vi "HFRR ADV v034 new software.vi"() -> ()   [LabVIEW 2025] (continued)
                      }
                      frame #22 {
                        n2405 = Wait (ms)(milliseconds to wait=u32 50) -> ()  [unwired: 1 out]
                      }
                      frame #23 {
                        n2406 = local read "NORMAL LOAD"() -> (w3468:dbl)
                        n2407 = Number To Fractional String(number=w3468, precision (6)=i16 2) -> (F-format string=w3469:string)  [unwired: 2 in]
                        n2408 = Concatenate Strings("Applied Load [grams] :" ("Content"), w3469) -> (w3471:string)
                        n2409 = local read "EVENT LOG"() -> (w3473:string)
                        n2410 = call "Event Log.vi"("Content"=w3471, "EVENT LOG"=w3473) -> ("EVENT LOG"=w3472:string)  [unwired: 8 in, 1 out]
                        n2411 = local write "EVENT LOG"(w3472) -> ()
                      }
                      frame #24 {
                        n2412 = Wait (ms)(milliseconds to wait=u32 50) -> ()  [unwired: 1 out]
                      }
                      frame #25 {
                        n2413 = local read "Set Strk"() -> (w3476:dbl)
                        n2414 = Number To Fractional String(number=w3476, precision (6)=i16 2) -> (F-format string=w3477:string)  [unwired: 2 in]
                        n2415 = Concatenate Strings("Set Stroke [mm] :" ("Content"), w3477) -> (w3479:string)
                        n2416 = local read "EVENT LOG"() -> (w3481:string)
                        n2417 = call "Event Log.vi"("Content"=w3479, "EVENT LOG"=w3481) -> ("EVENT LOG"=w3480:string)  [unwired: 8 in, 1 out]
                        n2418 = local write "EVENT LOG"(w3480) -> ()
                      }
                      frame #26 {
                        n2419 = Wait (ms)(milliseconds to wait=u32 50) -> ()  [unwired: 1 out]
                      }
                      frame #27 {
                        n2420 = local read "Set Temp"() -> (w3484:dbl)
                        n2421 = Number To Fractional String(number=w3484, precision (6)=i16 2) -> (F-format string=w3485:string)  [unwired: 2 in]
                        n2422 = Concatenate Strings("Set Temperature [deg C] :" ("Content"), w3485) -> (w3487:string)
                        n2423 = local read "EVENT LOG"() -> (w3489:string)
                        n2424 = call "Event Log.vi"("Content"=w3487, "EVENT LOG"=w3489) -> ("EVENT LOG"=w3488:string)  [unwired: 8 in, 1 out]
                        n2425 = local write "EVENT LOG"(w3488) -> ()
                      }
                      frame #28 {
                        n2426 = Wait (ms)(milliseconds to wait=u32 50) -> ()  [unwired: 1 out]
                      }
                      frame #29 {
                        n2427 = local read "Set Rh"() -> (w3492:dbl)
                        n2428 = Number To Fractional String(number=w3492, precision (6)=i16 2) -> (F-format string=w3493:string)  [unwired: 2 in]
                        n2429 = Concatenate Strings("Set Humidity [%RH] :" ("Content"), w3493) -> (w3495:string)
                        n2430 = local read "EVENT LOG"() -> (w3497:string)
                        n2431 = call "Event Log.vi"("Content"=w3495, "EVENT LOG"=w3497) -> ("EVENT LOG"=w3496:string)  [unwired: 8 in, 1 out]
                        n2432 = local write "EVENT LOG"(w3496) -> ()
                      }
                      frame #30 {
                        n2433 = Wait (ms)(milliseconds to wait=u32 50) -> ()  [unwired: 1 out]
                      }
                      frame #31 {
                        n2434 = local read "test time"() -> (w3500:dbl)
                        n2435 = Number To Fractional String(number=w3500, precision (6)=i16 1) -> (F-format string=w3501:string)  [unwired: 2 in]
                        n2436 = Concatenate Strings("Test Duration [mins] :" ("Content"), w3501) -> (w3503:string)
                        n2437 = local read "EVENT LOG"() -> (w3505:string)
                        n2438 = call "Event Log.vi"("Content"=w3503, "EVENT LOG"=w3505) -> ("EVENT LOG"=w3504:string)  [unwired: 8 in, 1 out]
                        n2439 = local write "EVENT LOG"(w3504) -> ()
                      }
                      frame #32 {
                        w3506 = dbl[] [] ("History Data")
                        w3507 = cluster{"y":dbl, dbl, "y":dbl}[] [] ("History Data")
                        w3508 = FALSE ("Visible")
                        n2440 = property on="Stroke ( mm )" class="WFChart (strict)"("History Data"=w3507) -> ()  [unwired: 2 in, 2 out]
                        n2441 = property on="Humidity ( %RH )" class="WFChart (strict)"("History Data"=w3506) -> ()  [unwired: 2 in, 2 out]
                        n2442 = property on="Temperature ( Deg C )" class="WFChart (strict)"("History Data"=w3506) -> ()  [unwired: 2 in, 2 out]
                        n2443 = property on="Electrical Contact Resistance ( % )" class="WFChart (strict)"("History Data"=w3506) -> ()  [unwired: 2 in, 2 out]
                        n2444 = property on="Coefficient of Friction" class="WFChart (strict)"("History Data"=w3506) -> ()  [unwired: 2 in, 2 out]
                        n2445 = property on="Frictional Force ( N )" class="WFChart (strict)"("History Data"=w3506) -> ()  [unwired: 2 in, 2 out]
                        n2446 = property on="Coefficient of Friction" class="WFChart (strict)"("History Data"=w3506) -> ()  [unwired: 2 in, 2 out]
                        n2447 = property on="Frictional Force ( N )" class="WFChart (strict)"("History Data"=w3506) -> ()  [unwired: 2 in, 2 out]
                        n2448 = property on="Electrical Contact Resistance ( % )" class="WFChart (strict)"("History Data"=w3506) -> ()  [unwired: 2 in, 2 out]
                        n2449 = property on="Humidity ( %RH )" class="WFChart (strict)"("History Data"=w3506) -> ()  [unwired: 2 in, 2 out]
                        n2450 = property on="Stroke ( mm )" class="WFChart (strict)"("History Data"=w3507) -> ()  [unwired: 2 in, 2 out]
                        n2451 = property on="Temperature ( Deg C )" class="WFChart (strict)"("History Data"=w3506) -> ()  [unwired: 2 in, 2 out]
                        n2452 = property on="Service Password Log" class="Str"("Visible"=w3508) -> ()  [unwired: 2 in, 2 out]
                        n2453 = property on="Password 3" class="Clust (strict)"("Visible"=w3508) -> ()  [unwired: 2 in, 2 out]
                      }
                    }
                    "TEST FILE NAM,E SAVED" <- TRUE ("TEST FILE NAM,E SAVED")
                  }
                }
              }
            }
          }
        }
        n2454 = local write "Test \nStatus"(w2889) -> ()
        n2455 = local write "Save"(w2889) -> ()
        n2456 = local read "Main Tab"() -> (w2883:T2)
        n2457 = case shown="True" w2886 {
          frame False {
            n2458 = local read "Rt 3"() -> (w2958:bool)
            n2459 = case shown="True" w2958 {
              frame False {
              }
              frame True {
                n2460 = local write "Rt 3"(FALSE ("Rt 3")) -> ()
              }
            }
            "Rt" <- TRUE ("Rt")
            "Rt 2" <- FALSE ("Rt")
          }
          frame True {
            n2461 = local read "Rt"() -> (w2964:bool)
            n2462 = local write "Rt 2"(TRUE ("Rt 2")) -> ()
            n2463 = case shown="True" w2964 {
              frame False {
              }
              frame True {
                n2464 = local write "Rt"(FALSE ("Rt")) -> ()
              }
            }
            "Rt 3" <- TRUE ("Rt 3")
          }
        }
        n2465 = case shown="Default" w2883 {
          tunnel: w2885 -> [_ w2993]
          frame Default {
            w2992 = 0.0 ("output")
            n2466 = local write "PID-out"(w2992) -> ()
            n2467 = local write "Frequency ( Hz )"(w2992) -> ()
            n2468 = local write "STROKE Initialize"(TRUE ("STROKE Initialize")) -> ()
          }
          frame "Acquire" {
            n2469 = stacked-sequence {
              frame #0 {
                n2470 = local read "Auto Start Test"() -> (w2995:bool)
                n2471 = case shown="True" w2995 {
                  tunnel: "RUN" -> [w3016 w3019]
                  tunnel: [w3016 w3018] -> w2996
                  frame False {
                  }
                  frame True {
                    n2472 = local read "Auto Start Temp"() -> (w3017:bool)
                    n2473 = Or(x=w3019, y=w3017) -> (x .or. y?=w3018:bool)
                  }
                }
                n2474 = local read "clk"() -> (w3015:dbl)
                n2475 = local read "Save"() -> (w3011:bool)
                n2476 = Equal?(x=w3015, y=0.0) -> (x = y?=w3012:bool)
                n2477 = And(x=w3012, y=w3011) -> (x .and. y?=w3013:bool)
                n2478 = Not(x="Engage") -> (.not. x?=w3002:bool)
                n2479 = case shown="False" w2996 {
                  tunnel: [0.0 w3042] -> w2998
                  frame False {
                    (unwired) TRUE ("Visible")
                    n2480 = local read "Auto Start Test"() -> (w3023:bool)
                    n2481 = local write "Start Time"(TRUE ("Start Time")) -> ()
                    n2482 = property on="Stroke 2" class="DigNum (strict)"("Visible"=FALSE) -> ()  [unwired: 2 in, 2 out]
                    n2483 = case shown="False" w3023 {
                      frame False {
                        n2484 = property on="Heater Button" class="Bool (strict)"("DisabledEnum"=T19."Enabled" ("Disabled")) -> ()  [unwired: 2 in, 2 out]
                        n2485 = property on="Humidity" class="Bool (strict)"("DisabledEnum"=T19."Enabled" ("Disabled")) -> ()  [unwired: 2 in, 2 out]
                      }
                      frame True {
                      }
                    }
                    n2486 = case shown="False" "TestCompFlg" {
                      frame False {
                        n2487 = local read "StartFlg"() -> (w3031:bool)
                        n2488 = case shown="True" w3031 {
                          frame False {
                          }
                          frame True {
                            n2489 = stacked-sequence {
                              frame #0 {
                                n2490 = local read "EVENT LOG"() -> (w3035:string)
                                n2491 = call "Event Log.vi"("Content"="Test was interrupted", "EVENT LOG"=w3035) -> ("EVENT LOG"=w3036:string)  [unwired: 8 in, 1 out]
                                n2492 = local write "EVENT LOG"(w3036) -> ()
                                n2493 = property on="RUN" class="Bool (strict)"("Visible"=TRUE) -> ()  [unwired: 2 in, 2 out]
                                n2494 = property on="Auto Start Test" class="Bool (strict)"("Visible"=TRUE) -> ()  [unwired: 2 in, 2 out]
                              }
                              frame #1 {
                                w3038 = FALSE ("StartFlg")
                                n2495 = property on="Heater Button" class="Bool (strict)"("Val(Sgnl)"=FALSE ("Value (Signaling)")) -> ()  [unwired: 2 in, 2 out]
                                n2496 = local write "Heater Button"(w3038) -> ()
                                n2497 = local write "StartFlg"(w3038) -> ()
                                n2498 = local write "Humidity"(w3038) -> ()
                              }
                              frame #2 {
                                n2499 = local write "Due Write"("VC;0" ("Command")) -> ()
                              }
                              frame #3 {
                                n2500 = Wait (ms)(milliseconds to wait=u32 1500) -> ()  [unwired: 1 out]
                              }
                              frame #4 {
                                n2501 = local write "Due Write"("HE;0" ("Command")) -> ()
                              }
                            }
                          }
                        }
                      }
                      frame True {
                      }
                    }
                    n2502 = local write "String 14"("Test will autostart once parameters reach the set value." ("String 14")) -> ()
                  }
                  frame True {
                    (unwired) FALSE ("Visible")
                    n2503 = property on="Stroke 2" class="DigNum (strict)"("Visible"=TRUE) -> ()  [unwired: 2 in, 2 out]
                    n2504 = property on="STOP 2" class="Bool (strict)"("Disabled"=u8 2) -> ()  [unwired: 2 in, 2 out]
                    n2505 = local write "String 14"(" Running....." ("String 14")) -> ()
                    n2506 = property on="Heater Button" class="Bool (strict)"("DisabledEnum"=T19."Disabled and Grayed Out" ("Disabled")) -> ()  [unwired: 2 in, 2 out]
                    n2507 = property on="Humidity" class="Bool (strict)"("DisabledEnum"=T19."Disabled and Grayed Out" ("Disabled")) -> ()  [unwired: 2 in, 2 out]
                    n2508 = case shown="True" "Start Time" {
                      selector: "Start Time" -> [_ w3061]
                      frame False {
                      }
                      frame True {
                        n2509 = Not(x=w3061) -> (.not. x?=w3060:bool)
                        n2510 = local write "Start Time"(w3060) -> ()
                        n2511 = local read "EVENT LOG"() -> (w3062:string)
                        n2512 = call "Event Log.vi"("Content"="Test in progress", "EVENT LOG"=w3062) -> ("EVENT LOG"=w3064:string)  [unwired: 8 in, 1 out]
                        n2513 = local write "EVENT LOG"(w3064) -> ()
                      }
                    }
                    n2514 = disable-structure shown="Enabled" {
                      disable-tunnel: [w3053 w3059] -> w3042
                      frame Disabled {
                        n2515 = local read "Set Hz"() -> (w3056:dbl)
                        n2516 = call <vilib>:"Uniform White Noise Waveform.vi"() -> ("signal out"=w3055:waveform(dbl))  [unwired: 10 in, 1 out]
                        n2517 = Random Number (0-1)() -> (number: 0 to 1=w3052:dbl)
                        n2518 = Add(x=w3056, y=w3055) -> (x+y=w3054:waveform(dbl))
                        n2519 = Multiply(x=ext 0.01 ("y"), y=w3052) -> (x*y=w3050:ext)
                        n2520 = Multiply(x=w3054, y=w3050) -> (x*y=w3053:waveform(ext))
                      }
                      frame Enabled {
                        n2521 = call-poly <vilib>:"Random Number (Range).vi"("lower bound (0)"=49.89, "upper bound (100)"=50.8) -> ("number"=w3059:dbl)  [unwired: 9 in]
                      }
                    }
                    "StartFlg" <- TRUE ("StartFlg")
                  }
                }
                n2522 = case shown="True" w3013 {
                  frame False {
                  }
                  frame True {
                    n2523 = local write "clk"(10.0 ("clk")) -> ()
                    n2524 = Get Date/Time In Seconds() -> (seconds since 1Jan1904=w3067:timestamp)
                    n2525 = To Double Precision Float(number=w3067) -> (double precision float=w3065:dbl)
                    n2526 = local write "acq timer"(w3065) -> ()
                    n2527 = local write "act save time"(w3065) -> ()
                  }
                }
                n2528 = call "Elapsed Time"("Time Target (s)"="Countdown", "Reset"=w3002) -> ("Elapsed Time (s)"=w3007:dbl, "Time has Elapsed"=w3005:bool)  [unwired: 10 in, 6 out]
                "Countdown 2" <- w3007
                n2529 = Subtract(x=w3007, y=2.0) -> (x-y=w3010:dbl)
                n2530 = Less?(x=w3010, y="Countdown") -> (x < y?=w3008:bool)
                n2531 = And(x=w3008, y=w3005) -> (x .and. y?=w3004:bool)
                n2532 = case shown="True" w3004 {
                  frame False {
                  }
                  frame True {
                    (unwired) dbl[] [] ("History Data")
                    n2533 = local write "Engage"(FALSE ("Engage")) -> ()
                    n2534 = local write "RUN"(TRUE ("RUN")) -> ()
                    n2535 = local read "Humidity ( %RH )"() -> (→"Rh Before":dbl)
                  }
                }
                n2536 = local read "Test \nStatus"() -> (w3000:bool)
                n2537 = Select(t=w2998, s=w3000, f=0.0) -> (s? t:f=w2999:dbl)
                n2538 = local write "Frequency ( Hz )"(w2999) -> ()
              }
              frame #1 {
                w3090 = 1000000.0 ("x")
                # "HC;1/0\nST;VALUE"
                # "Elapsed time\ncof\nstroke\nAir temp\nTemp\nHumidity"
                # "acq timer\n\nact save time"
                # "convert to microseconds"
                n2539 = local read "COUNT"() -> (w3073:i32)
                n2540 = local read "Rate"() -> (w3086:dbl)
                n2541 = Divide(x=w3090, y=w3086) -> (x/y=w3091:dbl)
                n2542 = Greater Or Equal?(x=w3073, y=250) -> (x >= y?=w3072:bool)
                n2543 = Get Date/Time In Seconds() -> (seconds since 1Jan1904=w3093:timestamp)
                n2544 = case shown="True" w3072 {
                  frame False {
                    n2545 = local read "COUNT"() -> (w3094:i32)
                    n2546 = Increment(x=w3094) -> (x+1=w3095:i32)
                    n2547 = local write "COUNT"(w3095) -> ()
                  }
                  frame True {
                    n2548 = local write "COUNT"(0 ("COUNT")) -> ()
                  }
                }
                n2549 = local read "Samplingtime 2"() -> (w3071:dbl)
                n2550 = local read "act save time"() -> (w3088:dbl)
                n2551 = Divide(x=w3091, y=w3090) -> (x/y=w3089:dbl)
                n2552 = To Double Precision Float(number=w3093) -> (double precision float=w3082:dbl)
                n2553 = Add(x=w3088, y=w3071) -> (x+y=w3087:dbl)
                n2554 = local read "acq timer"() -> (w3092:dbl)
                n2555 = local read "COUNT"() -> (w3075:i32)
                n2556 = Greater Or Equal?(x=w3082, y=w3087) -> (x >= y?=w3070:bool)
                n2557 = Multiply(x=w3089, y=w3075) -> (x*y=w3081:dbl)
                n2558 = Subtract(x=w3082, y=w3092) -> (x-y=w3084:dbl)
                n2559 = local read "Save"() -> (w3085:bool)
                n2560 = Add(x=w3084, y=w3081) -> (x+y=w3068:dbl)
                "Elapsed time 3" <- w3068
                n2561 = And(x=w3070, y=w3085) -> (x .and. y?=w3083:bool)
                n2562 = Divide(x=w3068, y=60.0) -> (x/y=w3079:dbl)
                n2563 = local read "Test \nStatus"() -> (w3069:bool)
                n2564 = local read "clk"() -> (w3076:dbl)
                n2565 = Equal?(x=w3076, y=10.0) -> (x = y?=w3078:bool)
                n2566 = case shown="True" w3083 {
                  tunnel: w3082 -> [_ w3208]
                  tunnel: [FALSE ("Boolean 2") TRUE ("Boolean 2")] -> _
                  frame False {
                  }
                  frame True {
                    w3162 = ";" ("Substring")
                    # "Pid out/\nFreq response value"
                    n2567 = local write "act save time"(w3208) -> ()
                    n2568 = local read "FILE"() -> (w3156:string)
                    n2569 = call "file check.vi"("file name in"=w3156) -> ("error out"=w3159:errorcluster, "file name out"=w3154:string)  [unwired: 9 in]
                    n2570 = local read "LVDT STROKE"() -> (w3151:dbl)
                    n2571 = local read "Add up Stroke"() -> (w3149:dbl)
                    n2572 = call "FILE PATH CREATION.vi"("error in"=w3159, "FILE NAME :"=w3154) -> ("FILE OUT"=w3157:path)  [unwired: 8 in, 1 out]
                    n2573 = local read "STROKE Initialize"() -> (w3144:bool)
                    n2574 = Concatenate Strings(w3154, ".dgf" ("Substring")) -> (w3158:string)
                    n2575 = Subtract(x=w3151, y=w3149) -> (x-y=w3150:dbl)
                    n2576 = Absolute Value(x=w3150) -> (abs(x)=w3147:dbl)
                    n2577 = local read "FF 2"() -> (→"Frictional Force ( N )" →"Frictional Force ( N )":dbl)
                    n2578 = Build Path(base path=w3157, name or relative path=w3158) -> (appended path=w3153:path)
                    n2579 = flat-sequence {
                      tunnel: w3147 -> [w3213]
                      tunnel: [w3212] -> w3145
                      tunnel: w3144 -> [w3210]
                      tunnel: [w3215] -> w3146
                      tunnel: w3145 -> [w3215]
                      frame #0 {
                        n2580 = call <vilib>:"Mean PtByPt.vi"("x"=w3213, "sample length"="STROKE FILTER", "initialize"=w3210) -> ("mean"=w3212:dbl)  [unwired: 1 in, 1 out]
                      }
                      frame #1 {
                        "STROKE Initialize" <- FALSE ("STROKE Initialize")
                      }
                    }
                    n2581 = local read "COF 2"() -> (w3167:dbl)
                    "Coefficient of Friction" <- w3167
                    "COF 4" <- w3167
                    "Coefficient of Friction" <- w3167
                    n2582 = local read "TEMP"() -> (w3170:dbl)
                    "Temperature ( Deg C )" <- w3170
                    n2583 = local read "Humidity ( %RH )"() -> (w3169:dbl)
                    "Humidity ( %RH )" <- w3169
                    "Humidity ( %RH )" <- w3169
                    n2584 = local read "Frequency ( Hz )"() -> (w3176:dbl)
                    n2585 = local read "LVDT STROKE DISPLAY"() -> (w3148:dbl)
                    n2586 = local read "Elapsed time"() -> (w3201:dbl)
                    n2587 = local read "AIR TEMP"() -> (w3174:dbl)
                    n2588 = local read "PID-out"() -> (w3179:dbl)
                    n2589 = local write "Temperature ( Deg C )"(w3170) -> ()
                    n2590 = Number To Fractional String(number=w3148, width (-)=i16 9 ("precision (6)"), precision (6)=i16 6) -> (F-format string=w3194:string)  [unwired: 1 in]
                    n2591 = Number To Fractional String(number=w3174, width (-)=i16 9 ("precision (6)"), precision (6)=i16 3) -> (F-format string=w3193:string)  [unwired: 1 in]
                    n2592 = Number To Fractional String(number=w3170, width (-)=i16 9 ("precision (6)"), precision (6)=i16 3) -> (F-format string=w3190:string)  [unwired: 1 in]
                    n2593 = Number To Fractional String(number=w3169, width (-)=i16 9 ("precision (6)"), precision (6)=i16 3) -> (F-format string=w3187:string)  [unwired: 1 in]
                    n2594 = Number To Fractional String(number=0.0, width (-)=i16 9 ("precision (6)"), precision (6)=i16 3) -> (F-format string=w3184:string)  [unwired: 1 in]
                    n2595 = Number To Fractional String(number=w3179, width (-)=i16 9 ("precision (6)"), precision (6)=i16 3) -> (F-format string=w3180:string)  [unwired: 1 in]
                    n2596 = Number To Fractional String(number=w3176, width (-)=i16 9 ("precision (6)"), precision (6)=i16 3) -> (F-format string=w3175:string)  [unwired: 1 in]
                    n2597 = Number To Fractional String(number=w3167, width (-)=i16 9 ("precision (6)"), precision (6)=i16 6) -> (F-format string=w3202:string)  [unwired: 1 in]
                    n2598 = Number To Fractional String(number=w3201, width (-)=i16 14 ("precision (6)"), precision (6)=i16 3) -> (F-format string=w3203:string)  [unwired: 1 in]
                    n2599 = Bundle("y"=1.02, "LVDT STROKE DISPLAY"=w3148, "y"=0.98) -> (w3168:T30)  [unwired: 1 in]
                    n2600 = Number To Fractional String(number="Ambient Humidity :", width (-)=i16 9 ("precision (6)"), precision (6)=i16 6) -> (F-format string=w3160:string)  [unwired: 1 in]
                    n2601 = local read "RUN"() -> (w3166:bool)
                    n2602 = case shown="True" w3166 {
                      tunnel: w3168 -> [_ w3219]
                      tunnel: w3148 -> [_ w3218]
                      tunnel: w3148 -> [_ w3216]
                      tunnel: w3148 -> [_ w3217]
                      frame False {
                      }
                      frame True {
                        "Stroke ( mm )" <- w3219
                        "Stroke ( mm )" <- w3219
                        "Stroke 4" <- w3218
                        "Stroke 3" <- w3216
                        "Stroke 2" <- w3217
                        "measured_stroke" <- w3216
                      }
                    }
                    n2603 = Concatenate Strings(w3203, w3162, w3202, w3162, w3194, w3162, w3193, w3162, w3190, w3162, w3187, w3162, w3184, w3162, w3180, w3162, w3175, w3162, w3160, "\r") -> (w3200:string)
                    n2604 = call <vilib>:"Write Characters To File.vi"("append to file? (new file:F)"=TRUE, "character string"=w3200, "file path (dialog if empty)"=w3153) -> ()  [unwired: 2 in, 1 out]
                    "refresh flag" <- TRUE ("refresh flag")
                    "LVDT STROKE Actual" <- w3146
                  }
                }
                n2605 = case shown="True" w3069 {
                  tunnel: w3079 -> [_ w3105]
                  tunnel: w3084 -> [_ w3115]
                  tunnel: [0.0 w3111] -> _
                  tunnel: w3078 -> [_ w3110]
                  tunnel: [0.0 w3109] -> _
                  tunnel: w3068 -> [_ w3109]
                  tunnel: w3082 -> [w3098 _]
                  frame False {
                    n2606 = local write "acq timer"(w3098) -> ()
                    n2607 = local write "Test Duration Status"(0.0 ("Test Duration Status")) -> ()
                  }
                  frame True {
                    n2608 = local read "Set Hz"() -> (w3112:dbl)
                    n2609 = local write "Elapsed time"(w3105) -> ()
                    n2610 = local read "test time"() -> (w3104:dbl)
                    n2611 = Multiply(x=w3115, y=w3112) -> (x*y=w3114:dbl)
                    n2612 = case shown="False" w3110 {
                      tunnel: w3114 -> [w3116 _]
                      tunnel: [w3116 1.0] -> w3111
                      frame False {
                        n2613 = local write "Cycles elapsed"(w3116) -> ()
                      }
                      frame True {
                      }
                    }
                    n2614 = Greater?(x=w3105, y=w3104) -> (0:w3113:bool)
                    n2615 = Subtract(x=w3104, y=w3105) -> (x-y=w3103:dbl)
                    n2616 = Multiply(x=w3103, y=60.0) -> (x*y=w3102:dbl)
                    n2617 = local write "Time Remaining"(w3102) -> ()
                    n2618 = local write "Remaining Time"(w3102) -> ()
                    n2619 = case shown="True" w3113 {
                      frame False {
                      }
                      frame True {
                        n2620 = stacked-sequence {
                          frame #0 {
                            w3121 = T19."Enabled" ("Disabled")
                            w3120 = FALSE ("TEST FILE NAM,E SAVED")
                            w3122 = "" ("FILE")
                            w3123 = TRUE ("Visible")
                            n2621 = local write "Humidity"(FALSE ("Humidity")) -> ()
                            n2622 = local write "RUN"(FALSE ("OK Button 2")) -> ()
                            n2623 = local write "Heater Button"(FALSE ("Heater Button")) -> ()
                            n2624 = local write "Auto Start Test"(FALSE ("Auto Start Test")) -> ()
                            n2625 = local write "TestCompFlg"(TRUE ("StpFlg")) -> ()
                            n2626 = local read "Humidity ( %RH )"() -> (→"Rh After":dbl)
                            n2627 = property on="STOP 2" class="Bool (strict)"("Disabled"=u8 0) -> ()  [unwired: 2 in, 2 out]
                            n2628 = local read "EVENT LOG"() -> (w3128:string)
                            n2629 = call "Event Log.vi"("Content"="Test Completed", "EVENT LOG"=w3128) -> ("EVENT LOG"=w3127:string)  [unwired: 8 in, 1 out]
                            n2630 = property on="RUN" class="Bool (strict)"("Visible"=w3123) -> ()  [unwired: 2 in, 2 out]
                            n2631 = property on="Auto Start Test" class="Bool (strict)"("Visible"=w3123) -> ()  [unwired: 2 in, 2 out]
                            n2632 = local write "Batch Ref Num :"(w3122) -> ()
                            n2633 = local write "FILE"(w3122) -> ()
                            n2634 = local write "EVENT LOG"(w3127) -> ()
                            n2635 = local write "TEST FILE NAM,E SAVED"(w3120) -> ()
                            n2636 = local write "Fuel Discription :"(w3122) -> ()
                            n2637 = local write "START TEMP"(w3120) -> ()
                            n2638 = local write "Remarks :"(w3122) -> ()
                            n2639 = local write "Main Dashboard Buttons"(T1."Imaging" ("Main Dashboard Buttons")) -> ()
                            n2640 = local write "Main Tab"(T2."Adv Scar" ("Main Tab")) -> ()
                            n2641 = property on="FRICVALZ 2" class="Bool (strict)"("DisabledEnum"=w3121) -> ()  [unwired: 2 in, 2 out]
                            n2642 = property on="FRICVALZ 3" class="Bool (strict)"("DisabledEnum"=w3121) -> ()  [unwired: 2 in, 2 out]
                            n2643 = property on="FRICVALZ 4" class="Bool (strict)"("DisabledEnum"=w3121) -> ()  [unwired: 2 in, 2 out]
                          }
                          frame #1 {
                            n2644 = Wait (ms)(milliseconds to wait=u32 1500) -> ()  [unwired: 1 out]
                          }
                          frame #2 {
                            n2645 = local write "Due Write"("VC;0") -> ()
                          }
                          frame #3 {
                            n2646 = Wait (ms)(milliseconds to wait=u32 1500) -> ()  [unwired: 1 out]
                          }
                          frame #4 {
                            n2647 = local write "Due Write"("VC;0") -> ()
                          }
                          frame #5 {
                            n2648 = Wait (ms)(milliseconds to wait=u32 1500) -> ()  [unwired: 1 out]
                          }
                          frame #6 {
                            n2649 = local write "Due Write"("ST;0") -> ()
                          }
                          frame #7 {
                            n2650 = local write "measured_stroke"(0.0 ("measured_stroke")) -> ()
                            n2651 = Wait (ms)(milliseconds to wait=u32 1500) -> ()  [unwired: 1 out]
                          }
                          frame #8 {
                            n2652 = local write "Due Write"("HE;0") -> ()
                          }
                        }
                      }
                    }
                    n2653 = Divide(x=w3105, y=w3104) -> (x/y=w3108:dbl)
                    n2654 = Multiply(x=w3108, y=100.0) -> (x*y=w3106:dbl)
                    n2655 = local write "Test Duration Status"(w3106) -> ()
                  }
                }
              }
              frame #2 {
                n2656 = case shown="True" "Heater Button" {
                  tunnel: [0.0 ("output") w3242] -> w3220
                  frame False {
                    w3223 = TRUE ("tmpchk")
                    n2657 = local read "TEMP"() -> (w3224:dbl)
                    n2658 = local write "Temp ini"(w3224) -> ()
                    n2659 = local write "Reset 4"(w3223) -> ()
                    n2660 = local write "tmpchk"(w3223) -> ()
                    n2661 = local write "reinit"(TRUE ("reinit")) -> ()
                    n2662 = local write "manual temp log"(TRUE ("manual temp log")) -> ()
                  }
                  frame True {
                    # "Logic to turn off\nthe heater when \ntemp is not rising.\nTime - 60 sec\nDelta t- 5°c"
                    n2663 = local read "Temp ini"() -> (w3231:dbl)
                    n2664 = local read "Auto Start Test"() -> (w3227:bool)
                    n2665 = Less?(x=w3231, y=53.0) -> (x < y?=w3229:bool)
                    n2666 = case shown="False" w3227 {
                      frame False {
                        n2667 = local read "Set Temp"() -> (w3251:dbl)
                        n2668 = local read "TEMP"() -> (w3250:dbl)
                        n2669 = Subtract(x=w3251, y=w3250) -> (x-y=w3249:dbl)
                        n2670 = Absolute Value(x=w3249) -> (abs(x)=w3248:dbl)
                        n2671 = Less?(x=w3248, y=0.5) -> (x < y?=w3246:bool)
                        n2672 = case shown="True" w3246 {
                          tunnel: "manual temp log" -> [_ w3252]
                          frame False {
                          }
                          frame True {
                            n2673 = case shown="True" w3252 {
                              selector: w3252 -> [_ w3253]
                              frame False {
                              }
                              frame True {
                                # "#Event log"
                                n2674 = Not(x=w3253) -> (.not. x?=w3254:bool)
                                n2675 = local write "manual temp log"(w3254) -> ()
                                n2676 = local read "EVENT LOG"() -> (w3257:string)
                                n2677 = call "Event Log.vi"("Content"="Target Temperature reached", "EVENT LOG"=w3257) -> ("EVENT LOG"=w3256:string)  [unwired: 8 in, 1 out]
                                n2678 = local write "EVENT LOG"(w3256) -> ()
                              }
                            }
                          }
                        }
                      }
                      frame True {
                        n2679 = local write "manual temp log"(TRUE ("manual temp log")) -> ()
                      }
                    }
                    n2680 = And(x="tmpchk", y=w3229) -> (x .and. y?=w3232:bool)
                    n2681 = case shown="True" w3232 {
                      frame False {
                      }
                      frame True {
                        n2682 = call "Elapsed Time8"("Time Target (s)"=300.0, "Reset"="Reset 4") -> ("Time has Elapsed"=w3259:bool)  [unwired: 10 in, 7 out]
                        n2683 = flat-sequence {
                          tunnel: w3259 -> [_]
                          frame #0 {
                            n2684 = local write "Reset 4"(FALSE ("Reset 4")) -> ()
                          }
                        }
                        n2685 = case shown="True" w3259 {
                          frame False {
                          }
                          frame True {
                            n2686 = local read "Temp ini"() -> (w3266:dbl)
                            n2687 = Add(x=w3266, y=5.0) -> (x+y=w3264:dbl)
                            n2688 = local read "TEMP"() -> (w3267:dbl)
                            n2689 = Greater?(x=w3267, y=w3264) -> (0:w3265:bool)
                            n2690 = case shown="False" w3265 {
                              frame False {
                                n2691 = local write "Heater Button"(FALSE ("Heater Button")) -> ()
                              }
                              frame True {
                                n2692 = local write "tmpchk"(FALSE ("tmpchk")) -> ()
                              }
                            }
                          }
                        }
                      }
                    }
                    n2693 = local read "Set Temp"() -> (w3240:dbl)
                    n2694 = local read "TEMP"() -> (w3234:dbl)
                    n2695 = call-poly <vilib>:"PID.vi"("reinitialize? (F)"="reinit", "dt (s)"=-1.0, "process variable"=w3234, "setpoint"=w3240) -> ("output"=w3237:dbl)  [unwired: 6 in, 1 out]
                    n2696 = Subtract(x=w3240, y=w3234) -> (x-y=w3241:dbl)
                    n2697 = Add(x=w3240, y=0.5) -> (x+y=w3238:dbl)
                    n2698 = Greater Or Equal?(x=w3234, y=w3238) -> ()  [unwired: 1 out]
                    n2699 = Select(t=0.0, s=FALSE, f=w3237) -> (s? t:f=w3236:dbl)
                    "PID output" <- w3236
                    n2700 = flat-sequence {
                      tunnel: w3236 -> [w3270]
                      tunnel: [w3270] -> w3242
                      frame #0 {
                        n2701 = local write "reinit"(FALSE ("reinit")) -> ()
                      }
                    }
                    n2702 = Bundle(w3241, "output"=w3236, "TEMP"=w3234) -> ()  [unwired: 1 in, 1 out]
                  }
                }
                "PID-out" <- w3220
              }
              frame #3 {
                n2703 = local read "TEMP"() -> (w3272:dbl)
                n2704 = Greater Or Equal?(x=w3272, y="Set Temp 2") -> (x >= y?=w3277:bool)
                n2705 = case shown="True" w3277 {
                  tunnel: [FALSE TRUE] -> w3275
                  frame False {
                  }
                  frame True {
                  }
                }
                "Status 13" <- w3275
                n2706 = And(x=w3275, y="trip1 8") -> (x .and. y?=w3274:bool)
                n2707 = case shown="True" w3274 {
                  frame False {
                    n2708 = local write "Heater Trip Temp"(TRUE ("Heater Trip Temp")) -> ()
                  }
                  frame True {
                    w3280 = FALSE ("OK Button 2")
                    n2709 = case shown="True" "Heater Trip Temp" {
                      selector: "Heater Trip Temp" -> [_ w3282]
                      frame False {
                      }
                      frame True {
                        n2710 = Not(x=w3282) -> (.not. x?=w3281:bool)
                        n2711 = local read "EVENT LOG"() -> (w3285:string)
                        n2712 = local write "Heater Trip Temp"(w3281) -> ()
                        n2713 = call "Event Log.vi"("Content"="Heater Trip", "EVENT LOG"=w3285) -> ("EVENT LOG"=w3284:string)  [unwired: 8 in, 1 out]
                        n2714 = local write "EVENT LOG"(w3284) -> ()
                      }
                    }
                    n2715 = local write "RUN"(w3280) -> ()
                    n2716 = property on="Auto Start Test" class="Bool (strict)"("Value"=w3280) -> ()  [unwired: 2 in, 2 out]
                    n2717 = local write "Heater Button"(w3280) -> ()
                  }
                }
              }
            }
            n2718 = case shown="False" w2993 {
              frame False {
                n2719 = disable-structure shown="Disabled" {
                  frame Disabled {
                    n2720 = stacked-sequence {
                      frame #0 {
                        n2721 = local write "RUN"(FALSE ("OK Button 2")) -> ()
                      }
                      frame #1 {
                      }
                    }
                  }
                  frame Enabled {
                  }
                }
              }
              frame True {
              }
            }
          }
        }
        n2722 = local read "Reset Graph"() -> (w2882:bool)
        n2723 = case shown="True" w2882 {
          selector: w2882 -> [_ w2899]
          frame False {
          }
          frame True {
            w2913 = 0.0 ("X Scale.Range:Maximum")
            n2724 = Not(x=w2899) -> (.not. x?=w2898:bool)
            n2725 = local write "Reset Graph"(w2898) -> ()
            n2726 = property on="Electrical Contact Resistance ( % )" class="WFChart (strict)"("XScale.Maximum"=600.0 ("X Scale.Range:Maximum"), "XScale.Minimum"=0.0 ("X Scale.Range:Minimum"), "YScale.Maximum"=100.0 ("Y Scale.Range:Maximum"), "YScale.Minimum"=0.0 ("Y Scale.Range:Minimum")) -> ()  [unwired: 2 in, 2 out]
            n2727 = property on="Frictional Force ( N )" class="WFChart (strict)"("XScale.Maximum"=600.0 ("X Scale.Range:Maximum"), "XScale.Minimum"=0.0 ("X Scale.Range:Minimum"), "YScale.Maximum"=100.0 ("Y Scale.Range:Maximum"), "YScale.Minimum"=0.0 ("Y Scale.Range:Minimum")) -> ()  [unwired: 2 in, 2 out]
            n2728 = property on="Temperature ( Deg C )" class="WFChart (strict)"("XScale.Maximum"=600.0 ("X Scale.Range:Maximum"), "XScale.Minimum"=0.0 ("X Scale.Range:Minimum"), "YScale.Maximum"=100.0 ("Y Scale.Range:Maximum"), "YScale.Minimum"=0.0 ("Y Scale.Range:Minimum")) -> ()  [unwired: 2 in, 2 out]
            n2729 = property on="Humidity ( %RH )" class="WFChart (strict)"("XScale.Maximum"=600.0 ("X Scale.Range:Maximum"), "XScale.Minimum"=0.0 ("X Scale.Range:Minimum"), "YScale.Maximum"=100.0 ("Y Scale.Range:Maximum"), "YScale.Minimum"=0.0 ("Y Scale.Range:Minimum")) -> ()  [unwired: 2 in, 2 out]
            n2730 = property on="Stroke ( mm )" class="WFChart (strict)"("XScale.Maximum"=600.0 ("X Scale.Range:Maximum"), "XScale.Minimum"=0.0 ("X Scale.Range:Minimum"), "YScale.Maximum"=100.0 ("Y Scale.Range:Maximum"), "YScale.Minimum"=0.0 ("Y Scale.Range:Minimum")) -> ()  [unwired: 2 in, 2 out]
            n2731 = property on="Coefficient of Friction" class="WFChart (strict)"("XScale.Maximum"=600.0 ("X Scale.Range:Maximum"), "XScale.Minimum"=0.0 ("X Scale.Range:Minimum"), "YScale.Maximum"=100.0 ("Y Scale.Range:Maximum"), "YScale.Minimum"=0.0 ("Y Scale.Range:Minimum")) -> ()  [unwired: 2 in, 2 out]
            n2732 = property on="Electrical Contact Resistance ( % )" class="WFChart (strict)"("XScale.Minimum"=0.0 ("X Scale.Range:Minimum"), "XScale.Maximum"=600.0 ("X Scale.Range:Maximum"), "YScale.Minimum"=0.0 ("Y Scale.Range:Minimum"), "YScale.Maximum"=100.0 ("Y Scale.Range:Maximum")) -> ()  [unwired: 2 in, 2 out]
            n2733 = property on="Temperature ( Deg C )" class="WFChart (strict)"("XScale.Minimum"=0.0 ("X Scale.Range:Minimum"), "XScale.Maximum"=600.0 ("X Scale.Range:Maximum"), "YScale.Minimum"=0.0 ("Y Scale.Range:Minimum"), "YScale.Maximum"=100.0 ("Y Scale.Range:Maximum")) -> ()  [unwired: 2 in, 2 out]
            n2734 = property on="Coefficient of Friction" class="WFChart (strict)"("XScale.Minimum"=0.0 ("X Scale.Range:Minimum"), "XScale.Maximum"=600.0 ("X Scale.Range:Maximum"), "YScale.Maximum"=1.0 ("X Scale.Range:Minimum"), "YScale.Minimum"=0.0 ("X Scale.Range:Minimum")) -> ()  [unwired: 2 in, 2 out]
            n2735 = property on="Frictional Force ( N )" class="WFChart (strict)"("XScale.Maximum"=600.0 ("X Scale.Range:Maximum"), "XScale.Minimum"=w2913, "YScale.Maximum"=10.0 ("Y Scale.Range:Maximum"), "YScale.Minimum"=w2913) -> ()  [unwired: 2 in, 2 out]
            n2736 = property on="Stroke ( mm )" class="WFChart (strict)"("XScale.Maximum"=600.0 ("X Scale.Range:Maximum"), "XScale.Minimum"=0.0 ("X Scale.Range:Minimum"), "YScale.Maximum"=100.0 ("Y Scale.Range:Maximum"), "YScale.Minimum"=0.0 ("Y Scale.Range:Minimum")) -> ()  [unwired: 2 in, 2 out]
            n2737 = property on="Humidity ( %RH )" class="WFChart (strict)"("XScale.Maximum"=600.0 ("X Scale.Range:Maximum"), "XScale.Minimum"=0.0 ("X Scale.Range:Minimum"), "YScale.Maximum"=100.0 ("Y Scale.Range:Maximum"), "YScale.Minimum"=0.0 ("Y Scale.Range:Minimum")) -> ()  [unwired: 2 in, 2 out]
          }
        }
      }
      frame "Compare Files" {
        # "Elapsed time\ncof\nstroke\nAir temp\nTemp\nHumidity"
        n2738 = case shown="True" "RSTV1 2" {
          frame False {
          }
          frame True {
            n2739 = property on="Humidity ( %RH )" class="XYGraph (strict)"("Y Scale.Display Format:Precision"=u8 0 ("Y Scale.Format & Precision:Precision")) -> ()  [unwired: 2 in, 2 out]
            n2740 = property on="Humidity ( %RH )" class="XYGraph (strict)"("X Scale.Range:Minimum"=0.0, "X Scale.Range:Maximum"=75.0, "Y Scale.Range:Minimum"=48.0, "Y Scale.Range:Maximum"=58.0) -> ()  [unwired: 2 in, 2 out]
          }
        }
        n2741 = case shown="True" "RST CP 2" {
          frame False {
          }
          frame True {
            n2742 = property on="XY Graph 13" class="XYGraph (strict)"("Y Scale.Display Format:Precision"=u8 0 ("Y Scale.Format & Precision:Precision")) -> ()  [unwired: 2 in, 2 out]
            n2743 = property on="XY Graph 13" class="XYGraph (strict)"("X Scale.Range:Minimum"=0.0, "X Scale.Range:Maximum"=75.0, "Y Scale.Range:Minimum"=0.0, "Y Scale.Range:Maximum"=100.0) -> ()  [unwired: 2 in, 2 out]
          }
        }
        n2744 = case shown="True" "RST CP" {
          frame False {
          }
          frame True {
            n2745 = property on="Sample Temperature ( °C )" class="XYGraph (strict)"("Y Scale.Display Format:Precision"=u8 2 ("Y Scale.Format & Precision:Precision")) -> ()  [unwired: 2 in, 2 out]
            n2746 = property on="Sample Temperature ( °C )" class="XYGraph (strict)"("X Scale.Range:Minimum"=0.0, "X Scale.Range:Maximum"=75.0, "Y Scale.Range:Minimum"=58.0, "Y Scale.Range:Maximum"=62.0) -> ()  [unwired: 2 in, 2 out]
          }
        }
        n2747 = case shown="True" "RSTV1 3" {
          frame False {
          }
          frame True {
            n2748 = property on="Air Temperature  ( °C )" class="XYGraph (strict)"("Y Scale.Display Format:Precision"=u8 2 ("Y Scale.Format & Precision:Precision")) -> ()  [unwired: 2 in, 2 out]
            n2749 = property on="Air Temperature  ( °C )" class="XYGraph (strict)"("X Scale.Range:Minimum"=0.0 ("Y Scale.Range:Minimum"), "X Scale.Range:Maximum"=75.0 ("Y Scale.Range:Maximum"), "Y Scale.Range:Minimum"=20.0 ("X Scale.Range:Minimum"), "Y Scale.Range:Maximum"=26.0 ("X Scale.Range:Maximum")) -> ()  [unwired: 2 in, 2 out]
          }
        }
        n2750 = case shown="True" "RSTV1 4" {
          frame False {
          }
          frame True {
            n2751 = property on="Stroke ( mm )" class="XYGraph (strict)"("Y Scale.Display Format:Precision"=u8 2 ("Y Scale.Format & Precision:Precision")) -> ()  [unwired: 2 in, 2 out]
            n2752 = property on="Stroke ( mm )" class="XYGraph (strict)"("X Scale.Range:Minimum"=0.0 ("Y Scale.Range:Maximum"), "X Scale.Range:Maximum"=75.0 ("X Scale.Range:Minimum"), "Y Scale.Range:Minimum"=0.98, "Y Scale.Range:Maximum"=1.02) -> ()  [unwired: 2 in, 2 out]
          }
        }
        n2753 = case shown="True" "rstv2" {
          frame False {
          }
          frame True {
            n2754 = property on="Coefficient Of Friction" class="XYGraph (strict)"("Y Scale.Display Format:Precision"=u8 3 ("Y Scale.Format & Precision:Precision")) -> ()  [unwired: 2 in, 2 out]
            n2755 = property on="Coefficient Of Friction" class="XYGraph (strict)"("X Scale.Range:Minimum"=0.0 ("Y Scale.Range:Maximum"), "X Scale.Range:Maximum"=75.0, "Y Scale.Range:Minimum"=0.0, "Y Scale.Range:Maximum"=1.0 ("X Scale.Range:Minimum")) -> ()  [unwired: 2 in, 2 out]
          }
        }
        n2756 = case shown="True" "RST CP 3" {
          frame False {
          }
          frame True {
            n2757 = property on="Air Temp ( °C ) vs Humidity ( % RH )" class="XYGraph (strict)"("X Scale.Range:Minimum"=18.0, "X Scale.Range:Maximum"=28.0 ("X Scale.Range:Minimum"), "Y Scale.Range:Minimum"=30.0 ("X Scale.Range:Minimum"), "Y Scale.Range:Maximum"=70.0 ("X Scale.Range:Minimum")) -> ()  [unwired: 2 in, 2 out]
          }
        }
        n2758 = case shown="True" "OPEN 1" {
          frame False {
          }
          frame True {
            (unwired) 0  # existing file
            w3561 = "Choose a datalog file to open"  # prompt
            n2759 = local write "OPEN 1"(FALSE ("OPEN 1")) -> ()
            n2760 = String To Path(string="C:\\LAB-IQ\\Data\\") -> (path=w3546:path)
            n2761 = File Dialog(6:"*.dgf" ("pattern"), 7:w3561, 11:w3546) -> (0:w3544:errorcluster, 3:w3552:path)  [unwired: 4 in, 2 out]
            n2762 = Unbundle(w3544) -> ()  [unwired: 3 out]
            n2763 = Strip Path(path=w3552) -> (name=w3551:string)  [unwired: 1 out]
            n2764 = Path To String(path=w3552) -> (string=w3547:string)
            "string1" <- w3547
            n2765 = Match Pattern(string=w3551, regular expression=".dgf") -> (before substring=→"String Control":string)  [unwired: 1 in, 3 out]
            n2766 = Match Pattern(string=w3547, regular expression=".dgf" ("substring (\"\")")) -> (before substring=w3557:string)  [unwired: 1 in, 3 out]
            n2767 = Concatenate Strings(w3557, ".duf" ("Substring")) -> (w3553:string)
            n2768 = String To Path(string=w3553) -> (path=w3558:path)
            n2769 = call <vilib>:"Read Characters From File.vi"("file path (dialog if empty)"=w3558, "start of read offset (chars.:0)"=60 ("start of read offset (chars.: 0)")) -> ("character string"=→"String Control 2":string)  [unwired: 4 in, 3 out]
          }
        }
        n2770 = case shown="True" "OPEN 2" {
          frame False {
          }
          frame True {
            (unwired) 0  # existing file
            w3579 = "Choose a datalog file to open"  # prompt
            n2771 = local write "OPEN 2"(FALSE ("OPEN 1")) -> ()
            n2772 = String To Path(string="C:\\LAB-IQ\\Data\\") -> (path=w3564:path)
            n2773 = File Dialog(6:"*.dgf" ("pattern"), 7:w3579, 11:w3564) -> (0:w3562:errorcluster, 3:w3570:path)  [unwired: 4 in, 2 out]
            n2774 = Unbundle(w3562) -> ()  [unwired: 3 out]
            n2775 = Strip Path(path=w3570) -> (name=w3568:string)  [unwired: 1 out]
            n2776 = Path To String(path=w3570) -> (string=w3565:string)
            "string1 2" <- w3565
            n2777 = Match Pattern(string=w3568, regular expression=".dgf") -> (before substring=→"String Control 3":string)  [unwired: 1 in, 3 out]
            n2778 = Match Pattern(string=w3565, regular expression=".dgf" ("substring (\"\")")) -> (before substring=w3576:string)  [unwired: 1 in, 3 out]
            n2779 = Concatenate Strings(w3576, ".duf" ("Substring")) -> (w3573:string)
            n2780 = String To Path(string=w3573) -> (path=w3571:path)
            n2781 = call <vilib>:"Read Characters From File.vi"("file path (dialog if empty)"=w3571, "start of read offset (chars.:0)"=60 ("start of read offset (chars.: 0)")) -> ("character string"=→"String Control 4":string)  [unwired: 4 in, 3 out]
          }
        }
        n2782 = case shown="True" "OPEN 3" {
          frame False {
          }
          frame True {
            (unwired) 0  # existing file
            w3597 = "Choose a datalog file to open"  # prompt
            n2783 = local write "OPEN 3"(FALSE ("OPEN 1")) -> ()
            n2784 = String To Path(string="C:\\LAB-IQ\\Data\\") -> (path=w3582:path)
            n2785 = File Dialog(6:"*.dgf" ("pattern"), 7:w3597, 11:w3582) -> (0:w3580:errorcluster, 3:w3588:path)  [unwired: 4 in, 2 out]
            n2786 = Unbundle(w3580) -> ()  [unwired: 3 out]
            n2787 = Strip Path(path=w3588) -> (name=w3586:string)  [unwired: 1 out]
            n2788 = Path To String(path=w3588) -> (string=w3583:string)
            "string1 3" <- w3583
            n2789 = Match Pattern(string=w3586, regular expression=".dgf") -> (before substring=→"String Control 5":string)  [unwired: 1 in, 3 out]
            n2790 = Match Pattern(string=w3583, regular expression=".dgf" ("substring (\"\")")) -> (before substring=w3593:string)  [unwired: 1 in, 3 out]
            n2791 = Concatenate Strings(w3593, ".duf" ("Substring")) -> (w3590:string)
            n2792 = String To Path(string=w3590) -> (path=w3594:path)
            n2793 = call <vilib>:"Read Characters From File.vi"("file path (dialog if empty)"=w3594, "start of read offset (chars.:0)"=60 ("start of read offset (chars.: 0)")) -> ("character string"=→"String Control 6":string)  [unwired: 4 in, 3 out]
          }
        }
        n2794 = case shown="True" "OPEN 4" {
          frame False {
          }
          frame True {
            (unwired) 0  # existing file
            w3615 = "Choose a datalog file to open"  # prompt
            n2795 = local write "OPEN 4"(FALSE ("OPEN 1")) -> ()
            n2796 = String To Path(string="C:\\LAB-IQ\\Data\\") -> (path=w3600:path)
            n2797 = File Dialog(6:"*.dgf" ("pattern"), 7:w3615, 11:w3600) -> (0:w3598:errorcluster, 3:w3606:path)  [unwired: 4 in, 2 out]
            n2798 = Unbundle(w3598) -> ()  [unwired: 3 out]
            n2799 = Strip Path(path=w3606) -> (name=w3604:string)  [unwired: 1 out]
            n2800 = Path To String(path=w3606) -> (string=w3601:string)
            "string1 4" <- w3601
            n2801 = Match Pattern(string=w3604, regular expression=".dgf") -> (before substring=→"String Control 7":string)  [unwired: 1 in, 3 out]
            n2802 = Match Pattern(string=w3601, regular expression=".dgf" ("substring (\"\")")) -> (before substring=w3611:string)  [unwired: 1 in, 3 out]
            n2803 = Concatenate Strings(w3611, ".duf" ("Substring")) -> (w3608:string)
            n2804 = String To Path(string=w3608) -> (path=w3612:path)
            n2805 = call <vilib>:"Read Characters From File.vi"("file path (dialog if empty)"=w3612, "start of read offset (chars.:0)"=60 ("start of read offset (chars.: 0)")) -> ("character string"=→"String Control 8":string)  [unwired: 4 in, 3 out]
          }
        }
      }
      frame "About" {
        # "Elapsed time\ncof\nstroke\nmean pos\nTemp\nHumidity"
        n2806 = disable-structure shown="Disabled" {
          frame Disabled {
            n2807 = case shown="True" "Export" {
              frame False {
              }
              frame True {
                w3637 = "                                      " ("string")
                w3639 = "\r"
                (unwired) i16 6 ("width (-)")
                w3716 = "\r"
                w3648 = "\r"
                n2808 = local write "Export"(FALSE ("Export")) -> ()
                n2809 = local read "String 29"() -> (w3685:string)
                n2810 = local read "String 34"() -> (w3673:string)
                n2811 = local read "String 35"() -> (w3668:string)
                n2812 = local read "String 37"() -> (w3664:string)
                n2813 = local read "String 36"() -> (w3661:string)
                n2814 = local read "String 38"() -> (w3658:string)
                n2815 = local read "String 39"() -> (w3655:string)
                n2816 = Match Pattern(string=w3685, regular expression=".dwm") -> (before substring=w3681:string)  [unwired: 1 in, 3 out]
                "before substring" <- w3681
                n2817 = local read "S 38"() -> (w3676:string)
                n2818 = local read "S 39"() -> (w3669:string)
                n2819 = local read "Temperature before test 2"() -> (w3705:dbl)
                n2820 = local read "Temperature after test 2"() -> (w3710:dbl)
                n2821 = local read "Humidity before test 2"() -> (w3691:dbl)
                n2822 = local read "Humidity after test 2"() -> (w3706:dbl)
                n2823 = local read "MWSD 2"() -> (w3702:dbl)
                n2824 = local read "WS1.4 2"() -> (w3718:dbl)
                n2825 = local read "HCF 2"() -> (w3714:dbl)
                n2826 = local read "AVP 2"() -> (w3703:dbl)
                n2827 = Concatenate Strings("1," ("string"), w3676) -> (w3675:string)
                n2828 = Concatenate Strings("2," ("string"), w3673) -> (w3672:string)
                n2829 = Concatenate Strings("3," ("string"), w3669) -> (w3671:string)
                n2830 = Concatenate Strings("4," ("string"), w3668) -> (w3667:string)
                n2831 = Concatenate Strings("5," ("string"), w3664) -> (w3665:string)
                n2832 = Concatenate Strings("6," ("string"), w3661) -> (w3662:string)
                n2833 = Concatenate Strings("7," ("string"), w3658) -> (w3659:string)
                n2834 = Concatenate Strings("8," ("string"), w3655) -> (w3656:string)
                n2835 = local read "Sample ID"() -> (w3723:string)
                n2836 = case shown="\"xlx\"" "Select File Type" {
                  tunnel: w3681 -> [w3726 w3728 w3730]
                  tunnel: [w3724 w3729 w3731] -> w3680
                  frame "xlx" {
                    n2837 = Concatenate Strings(w3726, ".xls" ("string")) -> (w3724:string)
                  }
                  frame "csv" {
                    n2838 = Concatenate Strings(w3728, ".csv" ("string")) -> (w3729:string)
                  }
                  frame "txt" {
                    n2839 = Concatenate Strings(w3730, ".txt" ("string")) -> (w3731:string)
                  }
                }
                n2840 = local read "Test Date"() -> (w3722:string)
                n2841 = local read "String 45"() -> (w3636:string)
                n2842 = local read "String 31"() -> (w3721:string)
                n2843 = local read "String 32"() -> (w3720:string)
                n2844 = local read "TITTLE"() -> (w3644:string)
                n2845 = Number To Fractional String(number=w3691, width (-)=i16 6, precision (6)=i16 2) -> (F-format string=w3690:string)  [unwired: 1 in]
                n2846 = Number To Fractional String(number=w3705, width (-)=i16 6, precision (6)=i16 2) -> (F-format string=w3711:string)  [unwired: 1 in]
                n2847 = Number To Fractional String(number=w3706, width (-)=i16 6, precision (6)=i16 2) -> (F-format string=w3704:string)  [unwired: 1 in]
                n2848 = Number To Fractional String(number=w3710, width (-)=i16 6, precision (6)=i16 2) -> (F-format string=w3709:string)  [unwired: 1 in]
                n2849 = Number To Fractional String(number=w3702, width (-)=i16 6, precision (6)=i16 2) -> (F-format string=w3700:string)  [unwired: 1 in]
                n2850 = Number To Fractional String(number=w3703, width (-)=i16 6, precision (6)=i16 2) -> (F-format string=w3701:string)  [unwired: 1 in]
                n2851 = Number To Fractional String(number=w3714, width (-)=i16 6, precision (6)=i16 2) -> (F-format string=w3715:string)  [unwired: 1 in]
                n2852 = Number To Fractional String(number=w3718, precision (6)=i16 2) -> (F-format string=w3719:string)  [unwired: 2 in]
                n2853 = local read "s.NO"() -> (w3638:string)
                n2854 = Concatenate Strings("=" ("string"), w3644) -> (w3643:string)
                n2855 = Concatenate Strings("S.No," ("string"), "                                       Parameters" ("string")) -> (w3649:string)
                n2856 = Concatenate Strings(w3716, w3675, w3690, w3716, w3672, w3711, w3716, w3671, w3704, w3716, w3667, w3709, w3716, w3665, w3700, w3716, w3662, w3701, w3716, w3659, w3715, w3716, w3656, w3719) -> (w3678:string)
                n2857 = Concatenate Strings(w3648, "," ("string"), w3636, w3638, w3637, w3720, w3723, w3637, w3721, w3722, w3648) -> (w3646:string)
                n2858 = local read "Tested by"() -> (w3652:string)
                n2859 = local read "String 33"() -> (w3653:string)
                n2860 = Concatenate Strings("," ("string"), "                                                                             " ("string")) -> (w3641:string)
                n2861 = Concatenate Strings(w3643, w3639, w3646, w3639, w3649, w3678, w3639, w3641, w3653, w3652) -> (→"export":string)
                n2862 = String To Path(string=w3680) -> (path=w3687:path)
                n2863 = local read "export"() -> (w3682:string)
                n2864 = call <vilib>:"Write Characters To File.vi"("append to file? (new file:F)"=FALSE, "character string"=w3682, "file path (dialog if empty)"=w3687) -> ()  [unwired: 2 in, 1 out]
              }
            }
          }
          frame Enabled {
          }
        }
        n2865 = case shown="True" "OK Button 17" {
          frame False {
          }
          frame True {
            (unwired) 0  # existing file
            w3940 = "Choose a datalog file to open"  # prompt
            n2866 = local write "OK Button 17"(FALSE ("OK Button 17")) -> ()
            n2867 = local read "String"() -> (w3935:string)
            n2868 = String To Path(string=w3935) -> (path=w3936:path)
            n2869 = File Dialog(6:"*.duf" ("pattern"), 7:w3940, 11:w3936) -> (0:w3927:errorcluster, 3:w3946:path)  [unwired: 4 in, 2 out]
            n2870 = Unbundle(w3927) -> ()  [unwired: 3 out]
            n2871 = Open/Create/Replace File "Open File"(file path (use dialog)=w3946) -> (refnum out=w3938:refnum<file>)  [unwired: 5 in, 2 out]
            n2872 = Strip Path(path=w3946) -> (name=w3944:string)  [unwired: 1 out]
            n2873 = Path To String(path=w3946) -> (string=w3929:string)
            n2874 = while {
              tunnel: w3938 -> [w3950]
              i -> [w3947]
              stop <- w3948 continue-if-true
              (unwired) TRUE ("line mode (F)")
              n2875 = Read from Text File "Read File"(file (use dialog)=w3950) -> (text=w3949:string)  [unwired: 3 in, 3 out]
              n2876 = local write "Numeric 16"(w3947) -> ()
              n2877 = String Length(string=w3949) -> (length=w3952:i32)
              n2878 = Greater?(x=w3952, y=1) -> (0:w3948:bool)
            }
            n2879 = local write "String 29"(w3929) -> ()
            n2880 = Search and Replace String(input string=w3929, search string=".duf", replace string=".dgf" ("replace string (\"\")")) -> (result string=→"String Indicator 4":string)  [unwired: 5 in, 3 out]
            n2881 = Match Pattern(string=w3944, regular expression=".dwm") -> (before substring=w3928:string)  [unwired: 1 in, 3 out]
            "String Indicator" <- w3928
            n2882 = Match Pattern(string=w3929, regular expression=".dwm" ("substring (\"\")")) -> (before substring=w3930:string)  [unwired: 1 in, 3 out]
            "String Indicator 3" <- w3930
            n2883 = local write "TITTLE 2"(w3928) -> ()
            n2884 = String To Path(string=w3930) -> (path=w3937:path)
            "path" <- w3937
            n2885 = call <vilib>:"Read Characters From File.vi"("file path (dialog if empty)"=w3937, "start of read offset (chars.:0)"=60 ("start of read offset (chars.: 0)")) -> ("character string"=→"String Indicator 2":string)  [unwired: 4 in, 3 out]
          }
        }
        n2886 = call <vilib>:"Query Available Printers.vi"() -> ("system configured printers"=w3629:string[])  [unwired: 9 in, 2 out]
        "System Configured Printers 2" <- w3629
        n2887 = local read "OK Button 16"() -> (w3626:bool)
        n2888 = case shown="True" "OK Button 16" {
          frame False {
          }
          frame True {
            n2889 = stacked-sequence {
              frame #0 {
